vi "PWM2 Stop.vi"(10 "ChannelIndex":u8, 11 "DevHandle":i32) -> (3 "function return":i32)   [LabVIEW 2010, in "usb2pwm.lvlib"]
doc: "int WINAPI PWM2_Stop(int DevHandle, unsigned char ChannelIndex);"
uses:
  usb2pwm.lvlib
  USB2XXX/trunk/USB2XXX/USB2XXX/vs2019/Release/USB2XXX.dll
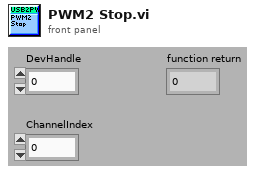
[diagram p1: front panel]
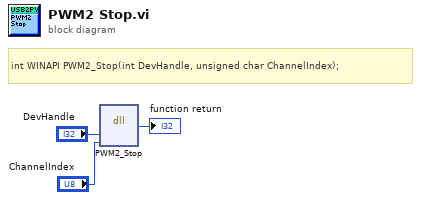
[diagram p0: block diagram]
diagram:
  # "int WINAPI PWM2_Stop(int DevHandle, unsigned char ChannelIndex);"
  n1 = dll-call lib="E:/Projects/USB2XXX/trunk/USB2XXX/USB2XXX/vs2019/Release/USB2XXX.*" fn="PWM2_Stop"("DevHandle"="DevHandle", "ChannelIndex"="ChannelIndex") -> (→"function return":i32)  [unwired: 5 in, 2 out]
